vi "Query Math Function Setting.vi"(8 "error in (no error)":errorcluster, 9 "Setting Type (0: Bin Size )":i32(ring) items=["Bin Size ", "Resolution Bandwidth", "Sample Rate"], 10 "Math Function Index (1: Math Function 1)":i32(ring)=1 items=["Math Function 1"=1, "Math Function 2"=2, "Math Function 3"=3, "Math Function 4"=4], 11 "VISA resource name":refnum<visa-resource-name>) -> (0 "error out":errorcluster, 2 "Setting Information":string, 3 "VISA resource name out":refnum<visa-resource-name>)   [LabVIEW 2015, in "Agilent 2000 3000 X-Series.lvlib"]
doc: "Returns the FFT function setting. \n\nNote:\nThis VI is not supported by EDUX1052A/G, DSOX1202A/G, DSOX1204A/G models."
uses:
  Agilent 2000 3000 X-Series.lvlib
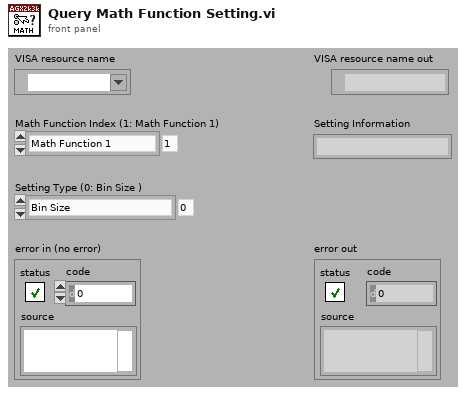
[diagram p1: front panel]
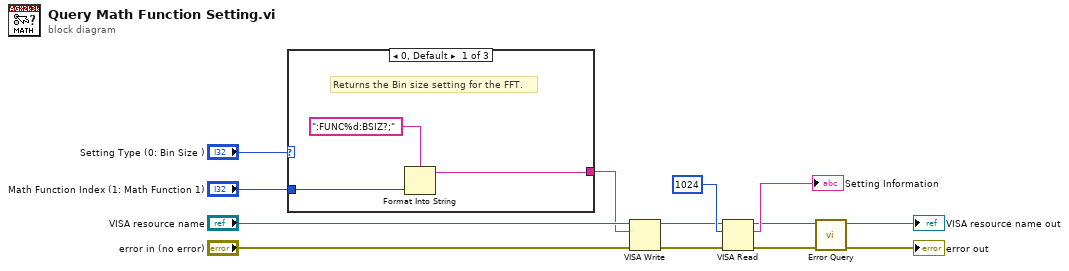
[diagram p0: block diagram]
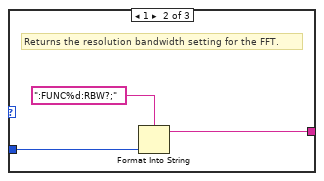
[diagram p2: hidden frame]
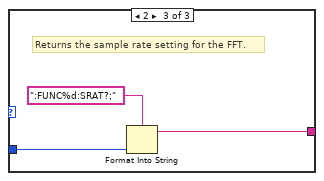
[diagram p3: hidden frame]
diagram:
  n1 = case shown="0, Default" "Setting Type (0: Bin Size )" {
    tunnel: "Math Function Index (1: Math Function 1)" -> [w15 w18 w21]
    tunnel: [w14 w17 w20] -> w6
    frame 0, Default {
      # "Returns the Bin size setting for the FFT."
      n2 = Format Into String(format string=":FUNC%d:BSIZ?;", w15) -> (resulting string=w14:string)  [unwired: 2 in, 1 out]
    }
    frame 1 {
      # "Returns the resolution bandwidth setting for the FFT."
      n3 = Format Into String(format string=":FUNC%d:RBW?;", w18) -> (resulting string=w17:string)  [unwired: 2 in, 1 out]
    }
    frame 2 {
      # "Returns the sample rate setting for the FFT."
      n4 = Format Into String(format string=":FUNC%d:SRAT?;", w21) -> (resulting string=w20:string)  [unwired: 2 in, 1 out]
    }
  }
  n5 = VISA Write(VISA resource name="VISA resource name", write buffer=w6, error in (no error)="error in (no error)") -> (VISA resource name out=w10:refnum<visa-resource-name>, error out=w9:errorcluster)  [unwired: 1 out]
  n6 = VISA Read(VISA resource name=w10, byte count=1024, error in (no error)=w9) -> (VISA resource name out=w4:refnum<visa-resource-name>, read buffer=→"Setting Information":string, error out=w3:errorcluster)  [unwired: 1 out]
  n7 = call "Error Query.vi"("error in (no error)"=w3, "VISA resource name"=w4) -> ("error out"=→"error out":errorcluster, "VISA resource name out"=→"VISA resource name out":refnum<visa-resource-name>)  [unwired: 6 in, 2 out]
